vi "실습 1-2.vi"() -> ()   [LabVIEW 2014]
uses:
  <vilib>/Analysis/NI_AALBase.lvlib
panel:
  in  "정지":bool
  out "웨이브폼 그래프":dbl[](graph)
  in  "사인파":bool
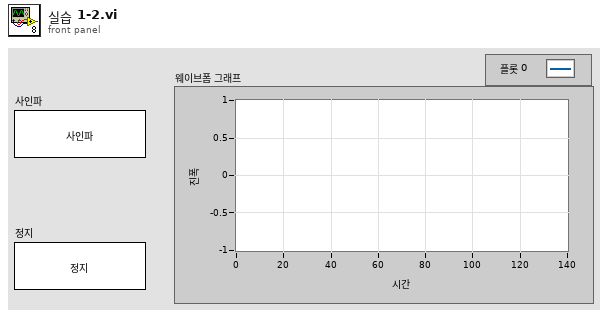
[diagram p1: front panel]
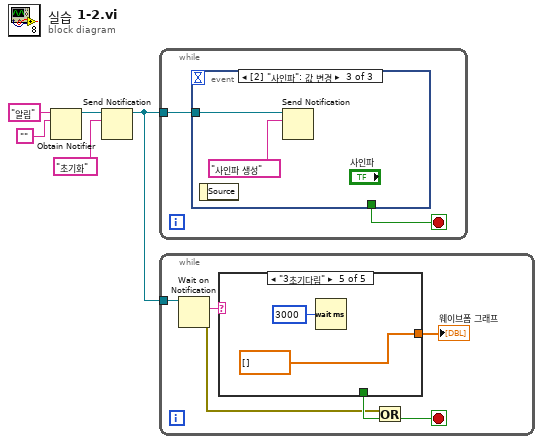
[diagram p0: block diagram]
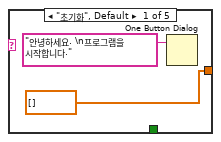
[diagram p2: hidden frame]
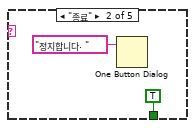
[diagram p3: hidden frame]
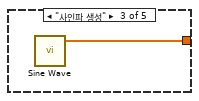
[diagram p4: hidden frame]
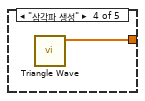
[diagram p5: hidden frame]
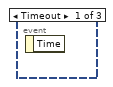
[diagram p6: hidden frame]
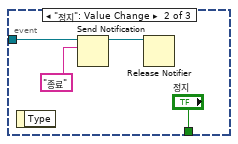
[diagram p7: hidden frame]
diagram:
  n1 = Obtain Notifier(name (unnamed)="알림" ("이름(이름없음)"), notification data type="") -> (notifier out=w5:refnum<notifier>)  [unwired: 2 in, 2 out]
  n2 = Send Notification(notification="초기화" ("알림"), notifier=w5) -> (notifier out=w1:refnum<notifier>)  [unwired: 1 in, 1 out]
  n3 = while {
    tunnel: w1 -> [w7]
    stop <- w6 stop-if-true
    n4 = event shown="[2] \"사인파\": 값 변경" {
      selector: _ -> [_ _ _]
      dyn-events: _ -> [_ _ _]
      timeout: _ -> [_ _ _]
      tunnel: w7 -> [_ w11 w13]
      tunnel: [_ "정지" _] -> w6
      event Timeout {
        n5 = event-data() -> ()  [unwired: 1 in, 1 out]
      }
      event "정지": Value Change {
        n6 = event-data() -> ()  [unwired: 1 in, 1 out]
        n7 = Send Notification(notification="종료" ("알림"), notifier=w11) -> (notifier out=w10:refnum<notifier>)  [unwired: 1 in, 1 out]
        n8 = Release Notifier(notifier=w10) -> ()  [unwired: 2 in, 3 out]
      }
      event "사인파": Value Change {
        n9 = event-data() -> ()  [unwired: 1 in, 1 out]
        n10 = Send Notification(notification="사인파 생성" ("알림"), notifier=w13) -> ()  [unwired: 1 in, 2 out]
      }
    }
  }
  n11 = while {
    tunnel: w1 -> [w19]
    stop <- w15 stop-if-true
    n12 = Wait on Notification(notifier=w19) -> (notification=w18:string, error out=w14:errorcluster)  [unwired: 3 in, 2 out]
    n13 = case shown="\"3초기다림\"" w18 {
      tunnel: [_ TRUE _ _ _] -> w17
      tunnel: [dbl[] [] ("웨이브폼 그래프") _ w24 w25 dbl[] [] ("웨이브폼 그래프")] -> w16
      frame "초기화", Default {
        n14 = One Button Dialog(message="안녕하세요. \n프로그램을 시작합니다." ("메시지")) -> ()  [unwired: 1 in, 1 out]
      }
      frame "종료" {
        n15 = One Button Dialog(message="정지합니다. " ("메시지")) -> ()  [unwired: 1 in, 1 out]
      }
      frame "사인파 생성" {
        n16 = call <vilib>:"Sine Wave.vi"() -> ("sine wave"=w24:dbl[])  [unwired: 5 in, 2 out]
      }
      frame "삼각파 생성" {
        n17 = call <vilib>:"Triangle Wave.vi"() -> ("triangle wave"=w25:dbl[])  [unwired: 5 in, 2 out]
      }
      frame "3초기다림" {
        n18 = Wait (ms)(milliseconds to wait=u32 3000 ("대기 시간(ms)")) -> ()  [unwired: 1 out]
      }
    }
    "웨이브폼 그래프" <- w16
    n19 = Or(x=w14, y=w17) -> (x .or. y?=w15:bool)
  }
